vi "gblVariable.vi"() -> ()   [LabVIEW 2020]
panel:
  in  "Status":refnum<vi>
  in  "Data Type":refnum<vi>
  in  "Item Type":refnum<vi>
  in  "Access Type":refnum<vi>
  in  "Delete":refnum<vi>
  in  "Add Field":refnum<vi>
  in  "Name":refnum<vi>
  in  "Records":refnum<vi>
  in  "Old Name":refnum<vi>
  in  "Old Tag":refnum<vi>
  in  "PV List":refnum<vi>
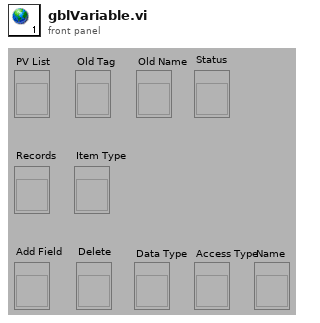
[diagram p1: front panel]
diagram:
